vi "StartEqualization.vi"(8 "error in (no error)":errorcluster, 11 "reference in":refnum<class "niMmWave_Reciever.lvclass">) -> (0 "error out":errorcluster, 2 "channel":T1, 3 "reference out":refnum<class "niMmWave_Reciever.lvclass">)   [LabVIEW 2019, in "niMmWave_Reciever.lvclass"]
doc: "Starts generating calibration pulse and prepares RX for acquisition"
uses:
  niMmWave_Reciever.lvclass
  C:/Barkhausen mmWave radar/Development/LV/Barkhausen mmWave hardware control/Host/SubVIs/mmWave instrument_class/mmWave instrument.lvclass
  mmWave instrument_class/Instrument state.ctl
  Low-level/TypeDefs/TX trigger config.ctl
  FPGA/SubVIs/Utility/FPGA driver trigger source.ctl
  FPGA/SubVIs/Utility/FPGA driver trigger destination.ctl
  <vilib>/Analysis/4window.llb/windowTd.ctl
  <vilib>/Analysis/1siggen.llb/Ramp Pattern by Samples.vi
  <vilib>/Analysis/2dsp.llb/Complex FFT.vi
  <vilib>/Analysis/baseanly.llb/Mean (DBL).vi
  <vilib>/Analysis/0measdsp.llb/Scaled Time Domain Window (CDB).vi
  <vilib>/Analysis/6fits.llb/1D B-Spline Fit.vi
  FPGA/SubVIs/Utility/FPGA Utility.lvlib
  mmWave HW Control/mmWave HW Control.lvlib
  <vilib>/Analysis/NI_AALBase.lvlib
  <vilib>/Analysis/NI_AALPro.lvlib
  mmWave instrument_class/mmWave instrument.lvclass
panel:
  out "magnitude":T2(graph)
  out "phase":T2(graph)
  out "Waveform Graph - Dark":dbl[][](graph)
  out "phase raw":cluster{"Ramp Pattern":dbl[], dbl[]}[](graph)
  out "magnitude raw":cluster{"Ramp Pattern":dbl[], dbl[]}[](graph)
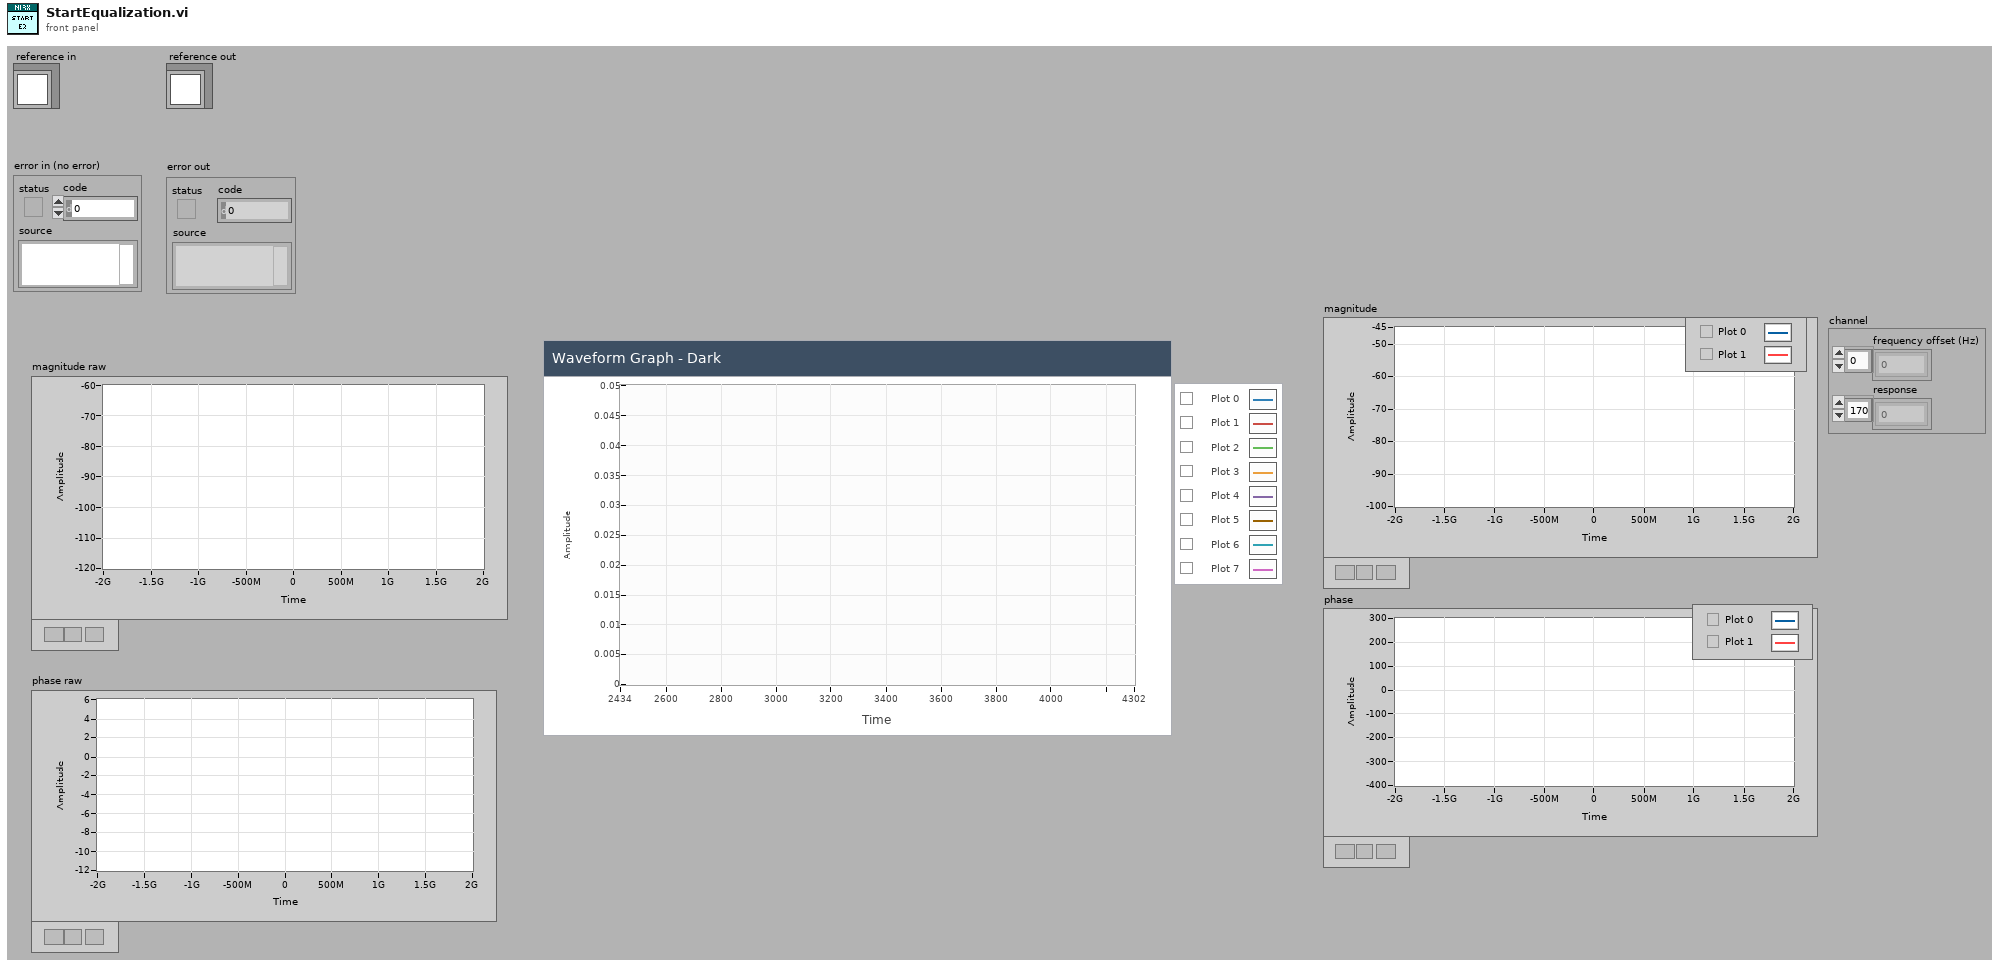
[diagram p1: front panel]
types:
  T1 = cluster{"frequency offset (Hz)":dbl[], "response":cdb[]}
  T2 = cluster{"Ramp Pattern":dbl[], "Best BSpline Fit Y":dbl[]}[]
  T3 = cluster{"frequency":u32, "gain":fxp<+/-,18,1>, "width":u8}
  T4 = typedef "mmWave instrument.lvclass/Instrument state.ctl" = enum16{"Off", "Initialization", "Configuration", "Running", "Calibration"}
  T5 = typedef "TX trigger config.ctl" = cluster{"delay":dbl, "trig source":T6, "PXI src":i32, "export":T7, "PXI dest":i32}
  T6 = typedef "FPGA Utility.lvlib/FPGA driver trigger source.ctl" = enum16{"Use Tclk", "PXI_Trig", "Aurora RX trig"}
  T7 = typedef "FPGA Utility.lvlib/FPGA driver trigger destination.ctl" = enum16{"None", "Source trig", "Synced trig", "Delayed sync"}
  T8 = typedef "niMmWave_Reciever.lvclass/ObjectAttributesRef.ctl" = refnum<data-value>
  T9 = typedef "niMmWave_Reciever.lvclass/ObjectAttributes.ctl" = cluster{"session":T10[], "HW.RX devices":T24, "RF config":T25, "RX trigger options":T5, "RX samples":i32, "RX Fs":dbl}
  T10 = typedef "Session.ctl" = cluster{"3620 session":refnum<queue>, "tx baseband session":T11, "rx baseband session":T19, "tx gain (dB)":dbl, "rx gain (dB)":dbl, "hardware configuration":T20, "gain ranging":T22[], "pxi trigger bus information":T23}
  T11 = typedef "Tx Baseband Session.ctl" = cluster{"3610 session":T12, "7902 reference":T18}
  T12 = typedef "ni3610_and_ni3630_Driver_Lib.lvlib/Main Settings.ctl" = cluster{"VISA resource name":refnum<visa-resource-name>, "Address Space":T13, "window_offset":u32, "register_addresses":T14, "required_MM_fpga_version":cluster{"signature":u32, "hardware":u32, "current revision":u32, "oldest revision":u32}, "CPLD Oldest Compat Version ":cluster{"hardware":u32, "CPLD firmware":u32}, "MM_FPGA_image_location":string, "is_init":bool, "card_type":T15, "DacLmkConfigFileName":string, "AdcLmkConfigFileName":string, "AdcConfigFileName":string, "DacConfigFileName_RevA":string, "DacConfigFileName_RevB":string, "Mulde hardware revision":u8, "bypass DAC PLL\n":bool, "IQ Card Revision":T16, "board capability":T17}
  T13 = typedef "VISA Register Access Address Space.ctl" = u16
  T14 = typedef "ni3610_and_ni3630_Driver_Lib.lvlib/Register Adresses.ctl" = cluster{"MM based Registers":cluster{"Revision":u32, "OldestCompatRev":u32, "signature":u32, "scratch":u32, "LedControl":u32, "BoardHwRev":u32, "BoardControl":u32, "ThermalStatus":u32, "BasebandStatus":u32, "BasebandControl":u32, "BasebandAuxSetup":u32, "BasebandAuxStatus":u32, "LmkSyncOutSetup":u32, " AdcSyncOutSetup":u32, " InjSyncOutSetup":u32, " PxiTrig0OutSetup":u32, " PxiTrig1OutSetup":u32, " PxiTrig2OutSetup":u32, " PxiTrig3OutSetup":u32, " PxiTrig4OutSetup":u32, " PxiTrig5OutSetup":u32, " PxiTrig6OutSetup":u32, " PxiTrig7OutSetup":u32}, "CPLD based Registers":cluster{"SlaveSignature":u32, "SlaveRevision":u32, "SlaveOldestCompatRev":u32, "SlaveScratch":u32, "SlaveSetup":u32, "SlaveStatus":u32, "IDacReg_offset":u32, "LMKRegGrp0_offset":u32, "QDacReg_offset":u32, "BrdTempSensorVal":u32, "TempSensorPowerDown":u32, "GPIOReg_offset":u32, "IAdcReg_offset":u32, "QAdcReg_offset":u32, "LMKRegGrp1_offset":u32, "QadcTempSensorVal":u32, "IadcTempSensorVal":u32, "RevisionReg":u32, "VcxoReg":u32, "CpldStatusReg":u32, "PowerReg":u32, "VBiasEnReg":u32, "ExtRefOeReg":u32, "QdacCtrlReg":u32, "QdacStatusReg":u32, "IdacCtrlReg":u32, "IdacStatusReg":u32, "QdacJtagIn":u32, "QdacJtagOut":u32, "IdacJtagIn":u32, "IdacJtagOut":u32, "IqDcSetupReg":u32, "QadcStatusReg":u32, "IadcStatusReg":u32, "BrdSetupReg":u32, "IqDcRevisionReg":u32, "PllStatusReg":u32, "EndpointScratchReg":u32, "AdcSyncCfgReg":u32, "IqCardOpampReg":u32}, "CPLD Register Offset":u32, "MM  Register Offset":u32, " PxiTrig0OutSetup":u32}
  T15 = typedef "ni3610_and_ni3630_Driver_Lib.lvlib/Base Card Type.ctl" = enum16{"unspecified", "ADC", "DAC"}
  T16 = typedef "ni3610_and_ni3630_Driver_Lib.lvlib/IQ Card Revision.ctl" = enum16{"RevA", "RevB", "RevC", "RevD"}
  T17 = typedef "ni3610_and_ni3630_Driver_Lib.lvlib/Board Capability.ctl" = cluster{"baseband sync":enum16{"no baseband sync", "baseband sync"}}
  T18 = typedef "Blank FPGA Reference.ctl" = refnum<k20>
  T19 = typedef "Rx Baseband Session.ctl" = cluster{"3630 session":T12, "7902 reference":T18}
  T20 = typedef "Hardware Configuration.ctl" = cluster{"direction":T21, "baseband only":bool}
  T21 = typedef "Direction.ctl" = enum16{"Transceiver", "Receiver", "Transmitter"}
  T22 = typedef "Gain Ranging.ctl" = cluster{"gain ranging active scope":string, "gain ranging stream session":refnum<k20>}
  T23 = typedef "PXI Trigger Bus Info.ctl" = cluster{"chassis resource name":refnum<visa-resource-name>, "7902R (TX)":i16, "3610 (TX)":i16, "3620 (IF)":i16, "3630 (RX)":i16, "7902R (RX)":i16}
  T24 = typedef "mmWave HW Control.lvlib/HW RX resources cluster.ctl" = cluster{"HW.IF":tag, "HW.ADC":refnum<visa-resource-name>, "HW.RX FPGA":tag}
  T25 = typedef "mmWave HW Control.lvlib/HW RX RF config cluster.ctl" = cluster{"Gain":dbl, "Frequency":dbl, "mmWave adapter":string}
  T26 = typedef "Constants.ctl" = cluster{"data clock rate (Hz)":dbl, "sample rate (Hz)":dbl, "sample rate selector string":string, "default tx bitfile path":path, "default rx bitfile path":path, "default proc bitfile path":path}
  T27 = typedef "NI_AALPro.lvlib/windowTd.ctl" = u32
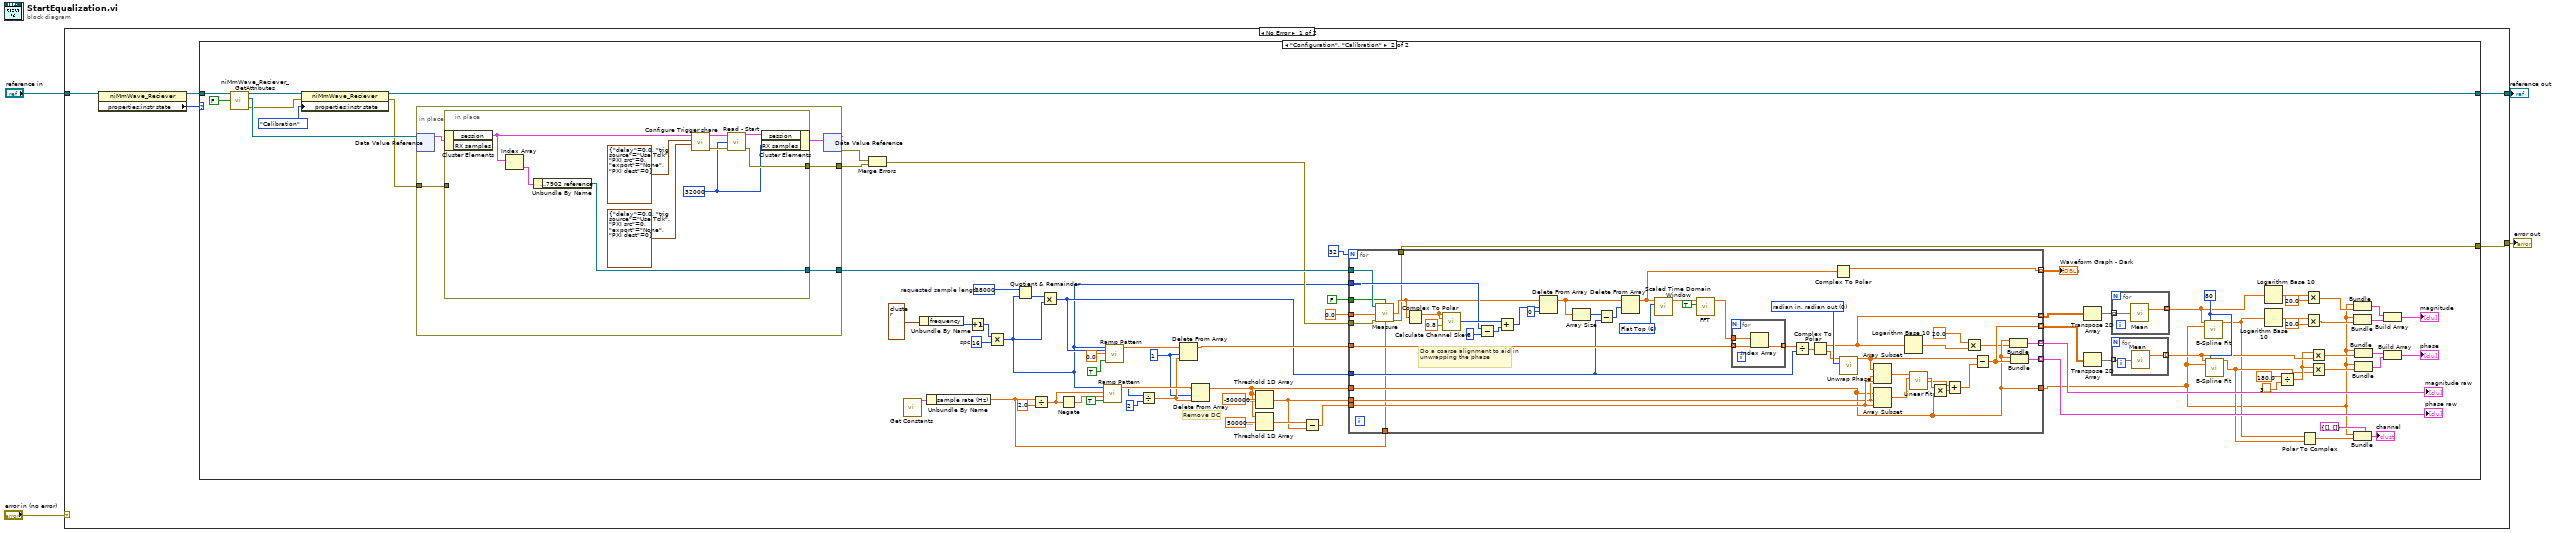
[diagram p0: block diagram]
diagram:
  n1 = case shown="No Error" "error in (no error)" {
    selector: "error in (no error)" -> [_ w158]
    tunnel: [w6 w158] -> w3
    tunnel: [w7 w157] -> w1
    tunnel: "reference in" -> [w9 w157]
    frame No Error {
      n2 = property class="niMmWave_Reciever"(reference=w9) -> (reference out=w8:refnum<class "niMmWave_Reciever.lvclass">, "properties:instr state"=w5:T4)  [unwired: 1 in, 1 out]
      n3 = case shown="\"Configuration\", \"Calibration\"" w5 {
        tunnel: w8 -> [w10 w86]
        tunnel: [w10 w77] -> w7
        tunnel: [_ w71] -> w6
        frame "Off", Default {
        }
        frame "Configuration", "Calibration" {
          w21 = 28000  # requested sample length
          w23 = 1 ("length")
          w20 = u32 16  # spc
          w62 = 80 ("# of control points")
          # "Remove DC"
          n4 = call "niMmWave_Reciever_GetAttributes.vi"("return data? (T)"=FALSE, "reference in"=w86) -> ("error out"=w40:errorcluster, "attributes ref"=w85:T8, "reference out"=w84:refnum<class "niMmWave_Reciever.lvclass">)  [unwired: 6 in, 1 out]
          n5 = property class="niMmWave_Reciever"(reference=w84, error in=w40, "properties:instr state"=Instrument_state."Calibration" ("instr state")) -> (reference out=w77:refnum<class "niMmWave_Reciever.lvclass">, error out=w39:errorcluster)
          n6 = in-place {
            in-place-border: w39 -> [w144]
            in-place-border: [w143] -> w83
            in-place-border: [w142] -> w75
            n7 = in-place-dvr #1(w85) -> (w146:T9)  [unwired: 1 out]
            n8 = in-place {
              in-place-border: w144 -> [_]
              in-place-border: [w149] -> w143
              in-place-border: [w147] -> w142
              w148 = u32 32000 ("number of samples")
              n9 = in-place-cluster #2(w146) -> ("session"=w155:T10[])  [unwired: 1 out]
              n10 = Index Array(array=w155) -> (element=w156:T10)  [unwired: 1 in]
              n11 = Unbundle By Name(w156) -> ("rx baseband session.7902 reference"=w147:T18)
              n12 = call "Configure Trigger share.vi"("RX trigger options"=T5 {"delay"=0.0, "trig source"=enum."Use Tclk", "PXI src"=0, "export"=enum."None", "PXI dest"=0} ("TX trigger options"), "TX trigger options"=T5 {"delay"=0.0, "trig source"=enum."Use Tclk", "PXI src"=0, "export"=enum."None", "PXI dest"=0}, "session in"=w155) -> ("error out"=w151:errorcluster, "session out"=w152:T10[])  [unwired: 5 in, 2 out]
              n13 = call "Read - Start.vi"("session in"=w152, "number of samples"=w148, "error in"=w151) -> ("session out"=w150:T10[], "error out"=w149:errorcluster)  [unwired: 11 in]
              n14 = in-place-cluster #2("session"=w150, "RX samples"=w148) -> (w145:T9)
            }
            n15 = in-place-dvr #1(w145) -> (w82:errorcluster)  [unwired: 1 out]
          }
          n16 = Merge Errors(w82, w83) -> (w72:errorcluster)
          n17 = call "Get Constants.vi"() -> ("constants"=w38:T26)  [unwired: 15 in]
          n18 = Unbundle By Name(T3 {"frequency"=10, "gain"=0.5, "width"=1} ("pulse parameters")) -> ("frequency"=w12:u32)
          n19 = Unbundle By Name(w38) -> ("sample rate (Hz)"=w11:dbl)
          n20 = Increment(x=w12) -> (x+1=w30:u32)
          n21 = Multiply(x=w30, y=w20) -> (x*y=w14:u32)
          n22 = Quotient & Remainder(x=w21, y=w14) -> (floor(x/y)=w36:u32)  [unwired: 1 out]
          n23 = Divide(x=w11, y=2.0) -> (x/y=w32:dbl)
          n24 = Multiply(x=w36, y=w14) -> (x*y=w15:u32)
          n25 = Negate(x=w32) -> (-x=w31:dbl)
          n26 = call-poly <vilib>:"Ramp Pattern.vi"("exclude end?"=TRUE, "start"=w31, "end"=w32, "samples"=w14) -> ("Ramp Pattern"=w35:dbl[])  [unwired: 6 in, 1 out]
          n27 = call-poly <vilib>:"Ramp Pattern.vi"("exclude end?"=TRUE, "start"=0.0, "end"=w15, "samples"=w14) -> ("Ramp Pattern"=w33:dbl[])  [unwired: 6 in, 1 out]
          n28 = Divide(x=w14, y=2) -> (x/y=w34:dbl)
          n29 = Delete From Array(array=w33, length=w23, index=w34) -> (array with subset deleted=w17:dbl[])  [unwired: 1 out]
          n30 = Delete From Array(array=w35, length=w23, index=w34) -> (array with subset deleted=w16:dbl[])  [unwired: 1 out]
          n31 = Threshold 1D Array(2:500000000.0 ("threshold y"), 3:w16) -> (0:w37:dbl)  [unwired: 1 in]
          n32 = Threshold 1D Array(2:-500000000.0 ("threshold y"), 3:w16) -> (0:w18:dbl)  [unwired: 1 in]
          n33 = Subtract(x=w37, y=w18) -> (x-y=w19:dbl)
          n34 = for {
            N: 32 -> [_]
            tunnel: [w116] -> w43 mode=indexing
            tunnel: w16 -> [w110]
            tunnel: w14 -> [w119]
            tunnel: [w110] -> w42
            tunnel: [w104] -> w44 mode=indexing
            tunnel: w17 -> [w128]
            tunnel: [w134] -> w81 mode=indexing
            tunnel: [w129] -> w80 mode=indexing
            tunnel: w15 -> [w118]
            tunnel: w19 -> [w112]
            tunnel: w18 -> [w111]
            tunnel: [w92] -> w78 mode=indexing
            tunnel: w75 -> [w99]
            tunnel: FALSE ("calculate measurements") -> [w98]
            tunnel: 0.0 ("frequency (Hz)") -> [w97]
            tunnel: w72 -> [w96]
            tunnel: w11 -> [w95]
            tunnel: [w93] -> w71
            w117 = T27 6 items=["Rectangle"=0, "Hanning"=1, "Hamming"=2, "Blackman-Harris"=3, "Exact Blackman"=4, "Blackman"=5, "Flat Top"=6, "4 Term B-Harris "=7, "7 Term B-Harris"=8, "Low Sidelobe"=9, "Blackman Nuttall"=11, "Triangle"=30, "Bartlett-Hanning"=31, "Bohman"=32, "Parzen"=33, "Welch"=34, "Kaiser"=60, "Dolph-Chebyshev"=61, "Gaussian"=62] ("window")
            w130 = 0 items=["radian in, radian out", "radian in, degree out", "degree in, degree out", "degree in, radian out"] ("phase unit")
            # "Do a coarse alignment to aid in unwrapping the phase"
            n35 = call "Measure.vi"("rx fpga reference in"=w99, "calculate measurements"=w98, "frequency (Hz)"=w97, "error in"=w96, "IQ rate"=w95) -> ("raw data"=w94:cdb[], "error out"=w93:errorcluster)  [unwired: 7 in, 2 out]
            n36 = Complex To Polar(r * e^(i*theta)=w94) -> (r=w121:dbl[])  [unwired: 1 out]
            n37 = call "Calculate Channel Skew.vi"("channel 1"=w121, "channel 2"=w121, "threshold"=0.8) -> ("falling edge index"=w126:i32)  [unwired: 10 in, 2 out]
            n38 = Subtract(x=w119, y=8) -> (x-y=w124:u32)
            n39 = Add(x=w126, y=w124) -> (x+y=w122:u32)
            n40 = Delete From Array(array=w94, length=w122, index=0) -> (array with subset deleted=w120:cdb[])  [unwired: 1 out]
            n41 = Array Size(array=w120) -> (size(s)=w137:i32)
            n42 = Subtract(x=w137, y=w118) -> (x-y=w136:u32)
            n43 = Delete From Array(array=w120, length=w136) -> (array with subset deleted=w100:cdb[])  [unwired: 1 in, 1 out]
            n44 = call-poly <vilib>:"Scaled Time Domain Window.vi"("window"=w117, "X"=w100) -> ("Windowed X"=w135:cdb[])  [unwired: 7 in, 2 out]
            n45 = call-poly <vilib>:"FFT.vi"("shift?"=TRUE, "X"=w135) -> ("FFT {X}"=w131:cdb[])  [unwired: 8 in, 1 out]
            n46 = for {
              tunnel: w128 -> [w141] mode=indexing
              tunnel: w131 -> [w140]
              tunnel: [w139] -> w133 mode=indexing
              n47 = Index Array(array=w140, index=w141) -> (element=w139:cdb)
            }
            n48 = Divide(x=w133, y=w118) -> (x/y=w132:cdb[])
            n49 = Complex To Polar(r * e^(i*theta)=w132) -> (r=w104:dbl[], theta=w105:dbl[])
            n50 = Complex To Polar(r * e^(i*theta)=w100) -> (r=w92:dbl[])  [unwired: 1 out]
            n51 = call <vilib>:"Unwrap Phase.vi"("phase unit"=w130, "Phase"=w105) -> ("Unwrapped Phase"=w115:dbl[])  [unwired: 8 in, 1 out]
            n52 = Array Subset(array=w115, index=w111, length=w112) -> (w114:dbl[])
            n53 = Array Subset(array=w110, index=w111, length=w112) -> (w113:dbl[])
            n54 = Logarithm Base 10(1:w104) -> (0:w103:dbl[])
            n55 = call <vilib>:"Linear Fit.vi"("Y"=w114, "X"=w113) -> ("slope"=w109:dbl, "intercept"=w107:dbl)  [unwired: 9 in, 3 out]
            n56 = Multiply(x=w109, y=w110) -> (x*y=w108:dbl[])
            n57 = Add(x=w107, y=w108) -> (x+y=w106:dbl[])
            n58 = Multiply(x=20.0, y=w103) -> (x*y=w101:dbl[])
            n59 = Subtract(x=w115, y=w106) -> (x-y=w116:dbl[])
            n60 = Bundle("Ramp Pattern"=w110, w101) -> (w134:cluster{"Ramp Pattern":dbl[], dbl[]})  [unwired: 1 in]
            n61 = Bundle("Ramp Pattern"=w110, w116) -> (w129:cluster{"Ramp Pattern":dbl[], dbl[]})  [unwired: 1 in]
          }
          "magnitude raw" <- w81
          "phase raw" <- w80
          "Waveform Graph - Dark" <- w78
          n62 = Transpose 2D Array(2D array=w44) -> (transposed array=w69:dbl[][])
          n63 = Transpose 2D Array(2D array=w43) -> (transposed array=w70:dbl[][])
          n64 = for {
            tunnel: w70 -> [w89] mode=indexing
            tunnel: [w88] -> w57 mode=indexing
            n65 = call-poly <vilib>:"Mean.vi"("X"=w89) -> ("mean"=w88:dbl)  [unwired: 1 out]
          }
          n66 = for {
            tunnel: w69 -> [w91] mode=indexing
            tunnel: [w90] -> w51 mode=indexing
            n67 = call-poly <vilib>:"Mean.vi"("X"=w91) -> ("mean"=w90:dbl)  [unwired: 1 out]
          }
          n68 = call-poly <vilib>:"B-Spline Fit.vi"("Y"=w51, "# of control points"=w62, "X"=w42) -> ("Best BSpline Fit Y"=w46:dbl[])  [unwired: 9 in, 3 out]
          n69 = call-poly <vilib>:"B-Spline Fit.vi"("Y"=w57, "# of control points"=w62, "X"=w42) -> ("Best BSpline Fit Y"=w54:dbl[])  [unwired: 9 in, 3 out]
          n70 = Logarithm Base 10(1:w51) -> (0:w50:dbl[])
          n71 = Logarithm Base 10(1:w46) -> (0:w47:dbl[])
          n72 = Divide(x=180.0, y=3.141592653589793) -> (x/y=w55:dbl)
          n73 = Polar To Complex(1:w54, 2:w46) -> (0:w61:cdb[])
          n74 = Multiply(x=w50, y=20.0) -> (x*y=w49:dbl[])
          n75 = Multiply(x=w47, y=20.0) -> (x*y=w45:dbl[])
          n76 = Multiply(x=w55, y=w57) -> (x*y=w56:dbl[])
          n77 = Multiply(x=w55, y=w54) -> (x*y=w53:dbl[])
          n78 = Bundle("Ramp Pattern"=w42, w49) -> (w68:cluster{"Ramp Pattern":dbl[], dbl[]})  [unwired: 1 in]
          n79 = Bundle("Ramp Pattern"=w42, w45) -> (w67:cluster{"Ramp Pattern":dbl[], dbl[]})  [unwired: 1 in]
          n80 = Bundle(cluster=T1 {"frequency offset (Hz)"=[], "response"=[]} ("channel 2"), "frequency offset (Hz)"=w42, "response"=w61) -> (→"channel":T1)
          n81 = Bundle("Ramp Pattern"=w42, w56) -> (w65:cluster{"Ramp Pattern":dbl[], dbl[]})  [unwired: 1 in]
          n82 = Bundle("Ramp Pattern"=w42, w53) -> (w64:cluster{"Ramp Pattern":dbl[], dbl[]})  [unwired: 1 in]
          n83 = Build Array(w68, w67) -> (→"magnitude":cluster{"Ramp Pattern":dbl[], dbl[]}[])
          n84 = Build Array(w65, w64) -> (→"phase":cluster{"Ramp Pattern":dbl[], dbl[]}[])
        }
      }
    }
    frame Error {
    }
  }
  "error out" <- w3
  "reference out" <- w1
